vi "Initialize.vi"(8 "error in (no error)":errorcluster {"code" format="%x"}, 10 "IP Address":u8[](array[numeric])=[192, 168, 10, 10], 11 "Comm Interface":T1) -> (0 "error out":errorcluster {"code" format="%x"})   [LabVIEW 2014, in "Keyence LK-G5000.lvlib"]
doc: "Establishes communication with the instrument and optionally performs an instrument identification query and/or an instrument reset. It also places the instrument in a default state needed for other instrument driver operations. Therefore, call this VI before calling other instrument driver VIs for this instrument. Generally, you need to call the Initialize VI only once at the beginning of an application."
uses:
  Keyence LK-G5000.lvlib
  Constant/Comm Interface.ctl
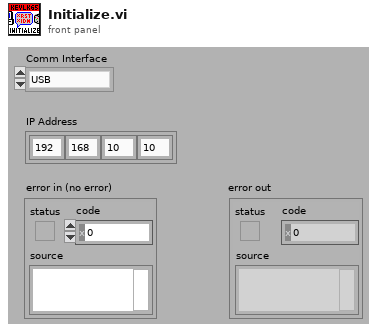
[diagram p1: front panel]
types:
  T1 = typedef "Keyence LK-G5000.lvlib/Comm Interface.ctl" = enum8{"USB", "ETHERNET"}
  T2 = cluster{"IP Address[0]":u8, "IP Address[1]":u8, "IP Address[2]":u8, "IP Address[3]":u8}
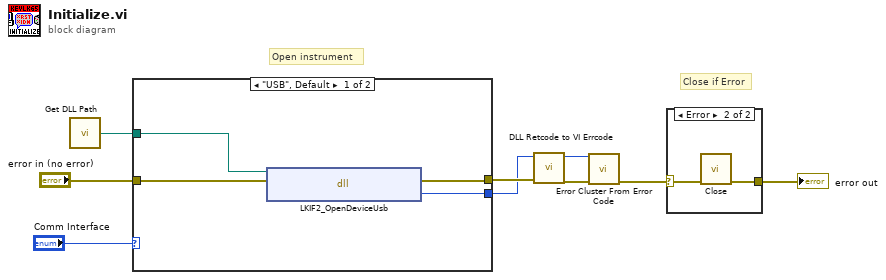
[diagram p0: block diagram]
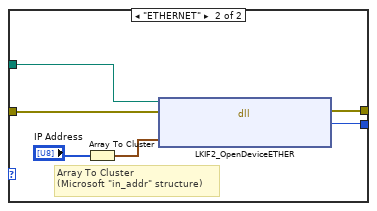
[diagram p3: hidden frame]
diagram:
  # "Close if Error"
  # "Open instrument"
  n1 = call "Get DLL Path.vi"() -> ("DLL Path"=w1:path)  [unwired: 1 in]
  n2 = case shown="\"USB\", Default" "Comm Interface" {
    tunnel: "error in (no error)" -> [w13 w19]
    tunnel: [w12 w18] -> w6
    tunnel: [w11 w17] -> w5
    tunnel: w1 -> [w10 w16]
    frame "USB", Default {
      n3 = dll-call lib="C:/Program Files/National Instruments/LabVIEW 2011/instr.lib/Keyence LK-G5000/LKIF2.dll" fn="LKIF2_OpenDeviceUsb"(path in=w10, error in=w13) -> (error out=w12:errorcluster, "RC"=w11:i32)  [unwired: 1 in, 1 out]
    }
    frame "ETHERNET" {
      # "Array To Cluster\n(Microsoft \"in_addr\" structure)"
      n4 = Array To Cluster(array="IP Address") -> (cluster=w14:T2)
      n5 = dll-call lib="C:/Program Files/National Instruments/LabVIEW 2011/instr.lib/Keyence LK-G5000/LKIF2.dll" fn="LKIF2_OpenDeviceETHER"(path in=w16, error in=w19, "OpenParam"=w14) -> (error out=w18:errorcluster, "RC"=w17:i32)  [unwired: 2 in, 1 out]
    }
  }
  n6 = call "DLL Retcode to VI Errcode.vi"("error in (no error)"=w6, "DLL Retcode"=w5) -> ("error out"=w4:errorcluster, "VI Errcode"=w3:i32)  [unwired: 8 in]
  n7 = call <vilib>:"Error Cluster From Error Code.vi"("error in (no error)"=w4, "error code (0)"=w3) -> ("error out"=w2:errorcluster)  [unwired: 7 in]
  n8 = case shown="Error" w2 {
    selector: w2 -> [w20 w21]
    tunnel: [w20 w22] -> w9
    frame No Error {
    }
    frame Error {
      n9 = call "Close.vi"("error in (no error)"=w21) -> ("error out"=w22:errorcluster)  [unwired: 10 in]
    }
  }
  "error out" <- w9
